vi "NI VeriStand - Get Macro Player Command Lines.vi"(8 "error in (no error)":errorcluster, 11 "MacroPlayer in":T3) -> (0 "error out":errorcluster, 2 "Command Lines":T1, 3 "MacroPlayer  out":T3)   [LabVIEW 2020, in "NI_VS MacroPlayerAPI.lvlib"]
doc: "Returns the commands the VeriStand Gateway sends to the RT target or desktop PC during recording. You must use the Open Command Line Notification (Macro Player) VI to open a reference to the command line of the Macro Player tool before you call this VI."
uses:
  <vilib>/NI VeriStand/Execution/MacroPlayer/NI_VS MacroPlayerAPI.lvlib
  <vilib>/NI VeriStand/Execution/MacroPlayer/MacroPlayerAPI.ctl
  NationalInstruments.VeriStand.ClientAPI
  <vilib>/NI VeriStand/Execution/MacroPlayer/Command Lines.ctl
  <vilib>/NI VeriStand/Execution/MacroPlayer/Command Line Info.ctl
  NationalInstruments.VeriStand.WorkspaceMacro
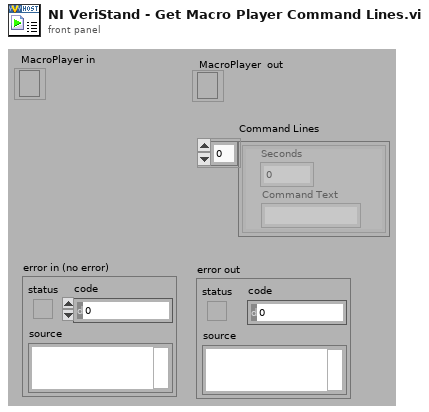
[diagram p1: front panel]
types:
  T1 = typedef "NI_VS MacroPlayerAPI.lvlib/Command Lines.ctl" = T2[]
  T2 = typedef "NI_VS MacroPlayerAPI.lvlib/Command Line Info.ctl" = cluster{"Seconds":dbl, "Command Text":string}
  T3 = typedef "NI_VS MacroPlayerAPI.lvlib/MacroPlayerAPI.ctl" = refnum<k24>
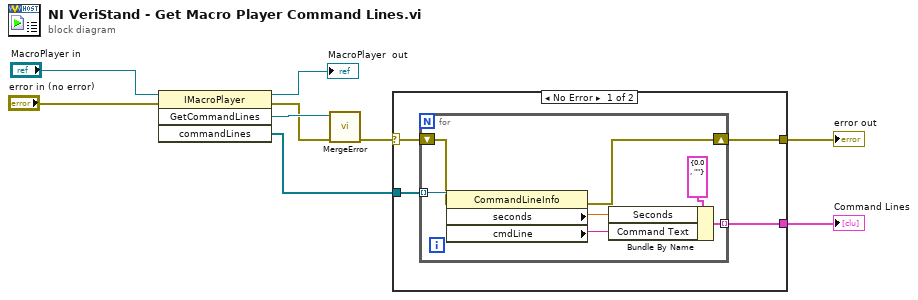
[diagram p0: block diagram]
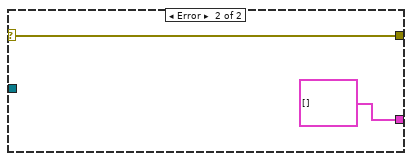
[diagram p2: hidden frame]
diagram:
  n1 = invoke class="IMacroPlayer" method="GetCommandLines"(reference="MacroPlayer in", error in="error in (no error)") -> (reference out=→"MacroPlayer  out":T3, error out=w4:errorcluster, "GetCommandLines"=w5:refnum<k24>, "commandLines"=w6:refnum<k24>[])  [unwired: 2 in]
  n2 = call <vilib>:"MergeError.vi"("error in (no error)"=w4, "Error"=w5) -> ("error out"=w2:errorcluster)  [unwired: 9 out]
  n3 = case shown="No Error" w2 {
    selector: w2 -> [w11 w21]
    tunnel: [w13 T2[] []] -> w7
    tunnel: w6 -> [w12 _]
    tunnel: [w10 w21] -> w1
    frame No Error {
      n4 = for {
        tunnel: w12 -> [w20] mode=indexing
        tunnel: [w16] -> w13 mode=indexing
        shift-right: [w14] -> w10
        shift-left: w11 -> [w15]
        n5 = property class="CommandLineInfo"(reference=w20, error in=w15) -> (error out=w14:errorcluster, "seconds"=w18:dbl, "cmdLine"=w17:string)  [unwired: 1 out]
        n6 = Bundle By Name(cluster=T2 {"Seconds"=0.0, "Command Text"=""} ("Macro Table Info"), "Seconds"=w18, "Command Text"=w17) -> (w16:T2)
      }
    }
    frame Error {
    }
  }
  "error out" <- w1
  "Command Lines" <- w7
